vi "mtlb simx Call Script Function a.vi"(5 "inBuffer":string, 6 "inString":string, 7 "inFloat":sgl, 8 "error in (no error)":errorcluster, 9 "inInt":i32, 10 "scriptDescriptionAndFunctionName":string, 11 "variousIntsIn":i32) -> (0 "error out":errorcluster, 3 "function return":i32)   [LabVIEW 2019, in "PXL_V-REP.lvlib"]
doc: "EXTAPI_DLLEXPORT simxInt mtlb_simxCallScriptFunction_a(const simxInt* variousIntsIn,const simxChar* scriptDescriptionAndFunctionName,const simxInt* inInt,const simxFloat* inFloat,const simxChar* inString,const simxUChar* inBuffer);"
uses:
  PXL_V-REP.lvlib
  <userlib>/V-REP/remoteApi.dll
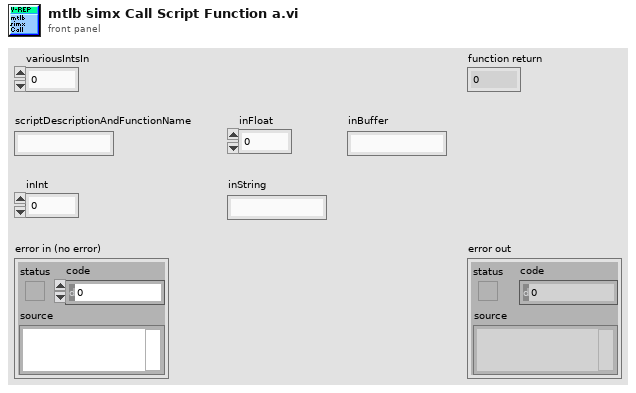
[diagram p1: front panel]
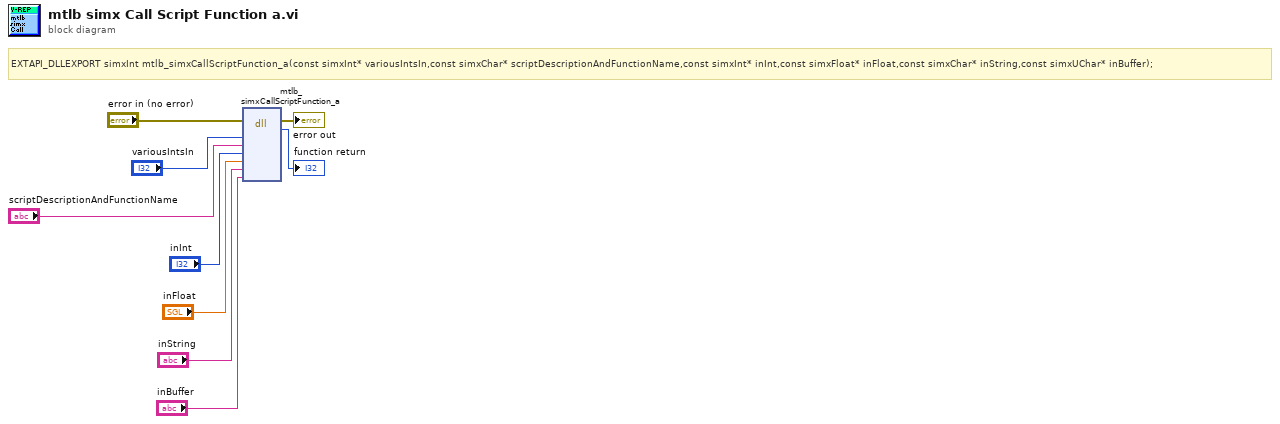
[diagram p0: block diagram]
diagram:
  # "EXTAPI_DLLEXPORT simxInt mtlb_simxCallScriptFunction_a(const simxInt* variousIntsIn,const simxChar* scriptDescriptionAndFunctionName,const simxInt* inInt,const simxFloat* inFloat,const simxChar* inString,const simxUChar* inBuffer);"
  n1 = dll-call lib="C:/Program Files (x86)/National Instruments/LabVIEW 2019/user.lib/V-REP/remoteApi.*" fn="mtlb_simxCallScriptFunction_a"(error in="error in (no error)", "variousIntsIn"="variousIntsIn", "scriptDescriptionAndFunctionName"="scriptDescriptionAndFunctionName", "inInt"="inInt", "inFloat"="inFloat", "inString"="inString", "inBuffer"="inBuffer") -> (error out=→"error out":errorcluster, →"function return":i32)  [unwired: 8 in, 1 out]
